vi "Generate File Header.vi"(11 "文件头数据":T1={"操作员姓名"="John Doe", "UUT序列号"="A001", "测试名称"="温度"}) -> (3 "文件头":string)   [LabVIEW 2012]
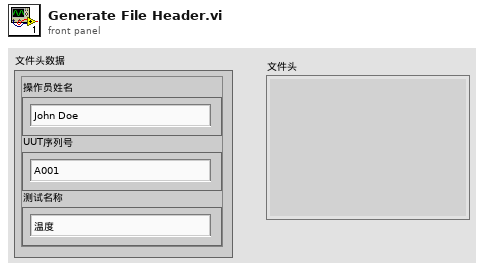
[diagram p1: front panel]
types:
  T1 = cluster{"操作员姓名":string, "UUT序列号":string, "测试名称":string}
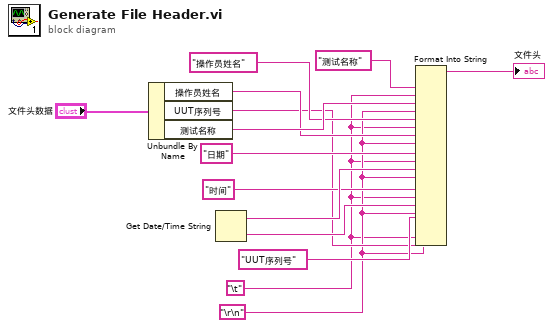
[diagram p0: block diagram]
diagram:
  w4 = "\r\n" ("行结束常量")
  w3 = "\t" ("制表符常量")
  n1 = Unbundle By Name ("按名称解除捆绑")("文件头数据") -> ("操作员姓名"=w11:string, "UUT序列号"=w5:string, "测试名称"=w13:string)
  n2 = Get Date/Time String ("获取日期/时间字符串")() -> (date string=w9:string, time string=w7:string)  [unwired: 3 in]
  n3 = Format Into String ("格式化写入字符串")("测试名称", w3, w13, w4, "操作员姓名", w3, w11, w4, "日期", w3, w9, w4, "时间", w3, w7, w4, "UUT序列号", w3, w5, w4) -> (resulting string=→"文件头":string)  [unwired: 3 in, 1 out]
